vi "MedicionAmplitud&Frecuencia.vi"(11 "data":dbl[](array[numeric])) -> (3 "Channel":T1)   [LabVIEW 2019, in "Prueba33.lvclass"]
uses:
  Prueba33.lvclass
  <vilib>/measure/mascope.llb/Amplitude and Levels 1 chan.vi
  <vilib>/measure/matone.llb/Harmonic Distortion Analyzer 1 Chan.vi
  <vilib>/measure/NI_MAPro.lvlib
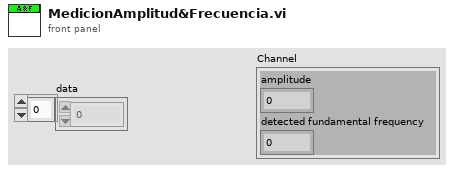
[diagram p1: front panel]
types:
  T1 = cluster{"amplitude":dbl, "detected fundamental frequency":dbl}
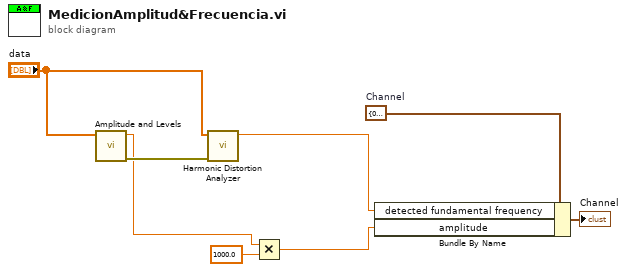
[diagram p0: block diagram]
diagram:
  w6 = T1 {"amplitude"=0.0, "detected fundamental frequency"=0.0}  # Channel
  n1 = call-poly <vilib>:"Amplitude and Levels.vi"("signal in"="data") -> ("error out"=w7:errorcluster, "amplitude"=w2:dbl)  [unwired: 7 in, 2 out]
  n2 = call-poly <vilib>:"Harmonic Distortion Analyzer.vi"("error in (no error)"=w7, "signal in"="data") -> ("detected fundamental frequency"=w5:dbl)  [unwired: 4 in, 5 out]
  n3 = Multiply(x=w2, y=1000.0) -> (x*y=w1:dbl)
  n4 = Bundle By Name(cluster=w6, "detected fundamental frequency"=w5, "amplitude"=w1) -> (→"Channel":T1)
